vi "Calcudavidflores.vi"() -> ()   [LabVIEW 2018]
uses:
  <vilib>/gmath/NI_Gmath.lvlib
panel:
  out "Ope 3":string
  in  "Numeric":u8
  out "Ope":string
  out "Display 2":string
  out "Ope 2":string
  out "Display":string
  in  "Cluster":T1={"Btn x^2"=FALSE, "Btn Tan -1 3"=FALSE, "Btn Tan -1 2"=FALSE, "Btn ."=FALSE, "Btn 8"=FALSE, "Btn 9"=FALSE, "Btn 7"=FALSE, "Btn 6"=FALSE, "Btn 5"=FALSE, "Btn 4"=FALSE, "Btn 3"=FALSE, "Btn 2"=FALSE, "Btn 1"=FALSE, "Btn 0"=FALSE, "Btn /"=FALSE, "Btn *"=FALSE, "Btn -"=FALSE, "Btn +"=FALSE, "Btn Tan -1"=FALSE, "Btn Cos-1"=FALSE, "Btn Sen -1"=FALSE, "Btn Sqrt"=FALSE, "Btn log"=FALSE, "Btn Tan"=FALSE, "Btn Cos"=FALSE, "Btn Sen"=FALSE, "Btn ="=FALSE, "Btn AC"=FALSE, "Btn Graf"=FALSE, "Btn e^x"=FALSE, "Btn X"=FALSE, "Bot Graficar"=TRUE, "btn grados"=FALSE, "btn radianes"=FALSE}
  out "Display_Calculadora":string
  in  "Display_Graf":string
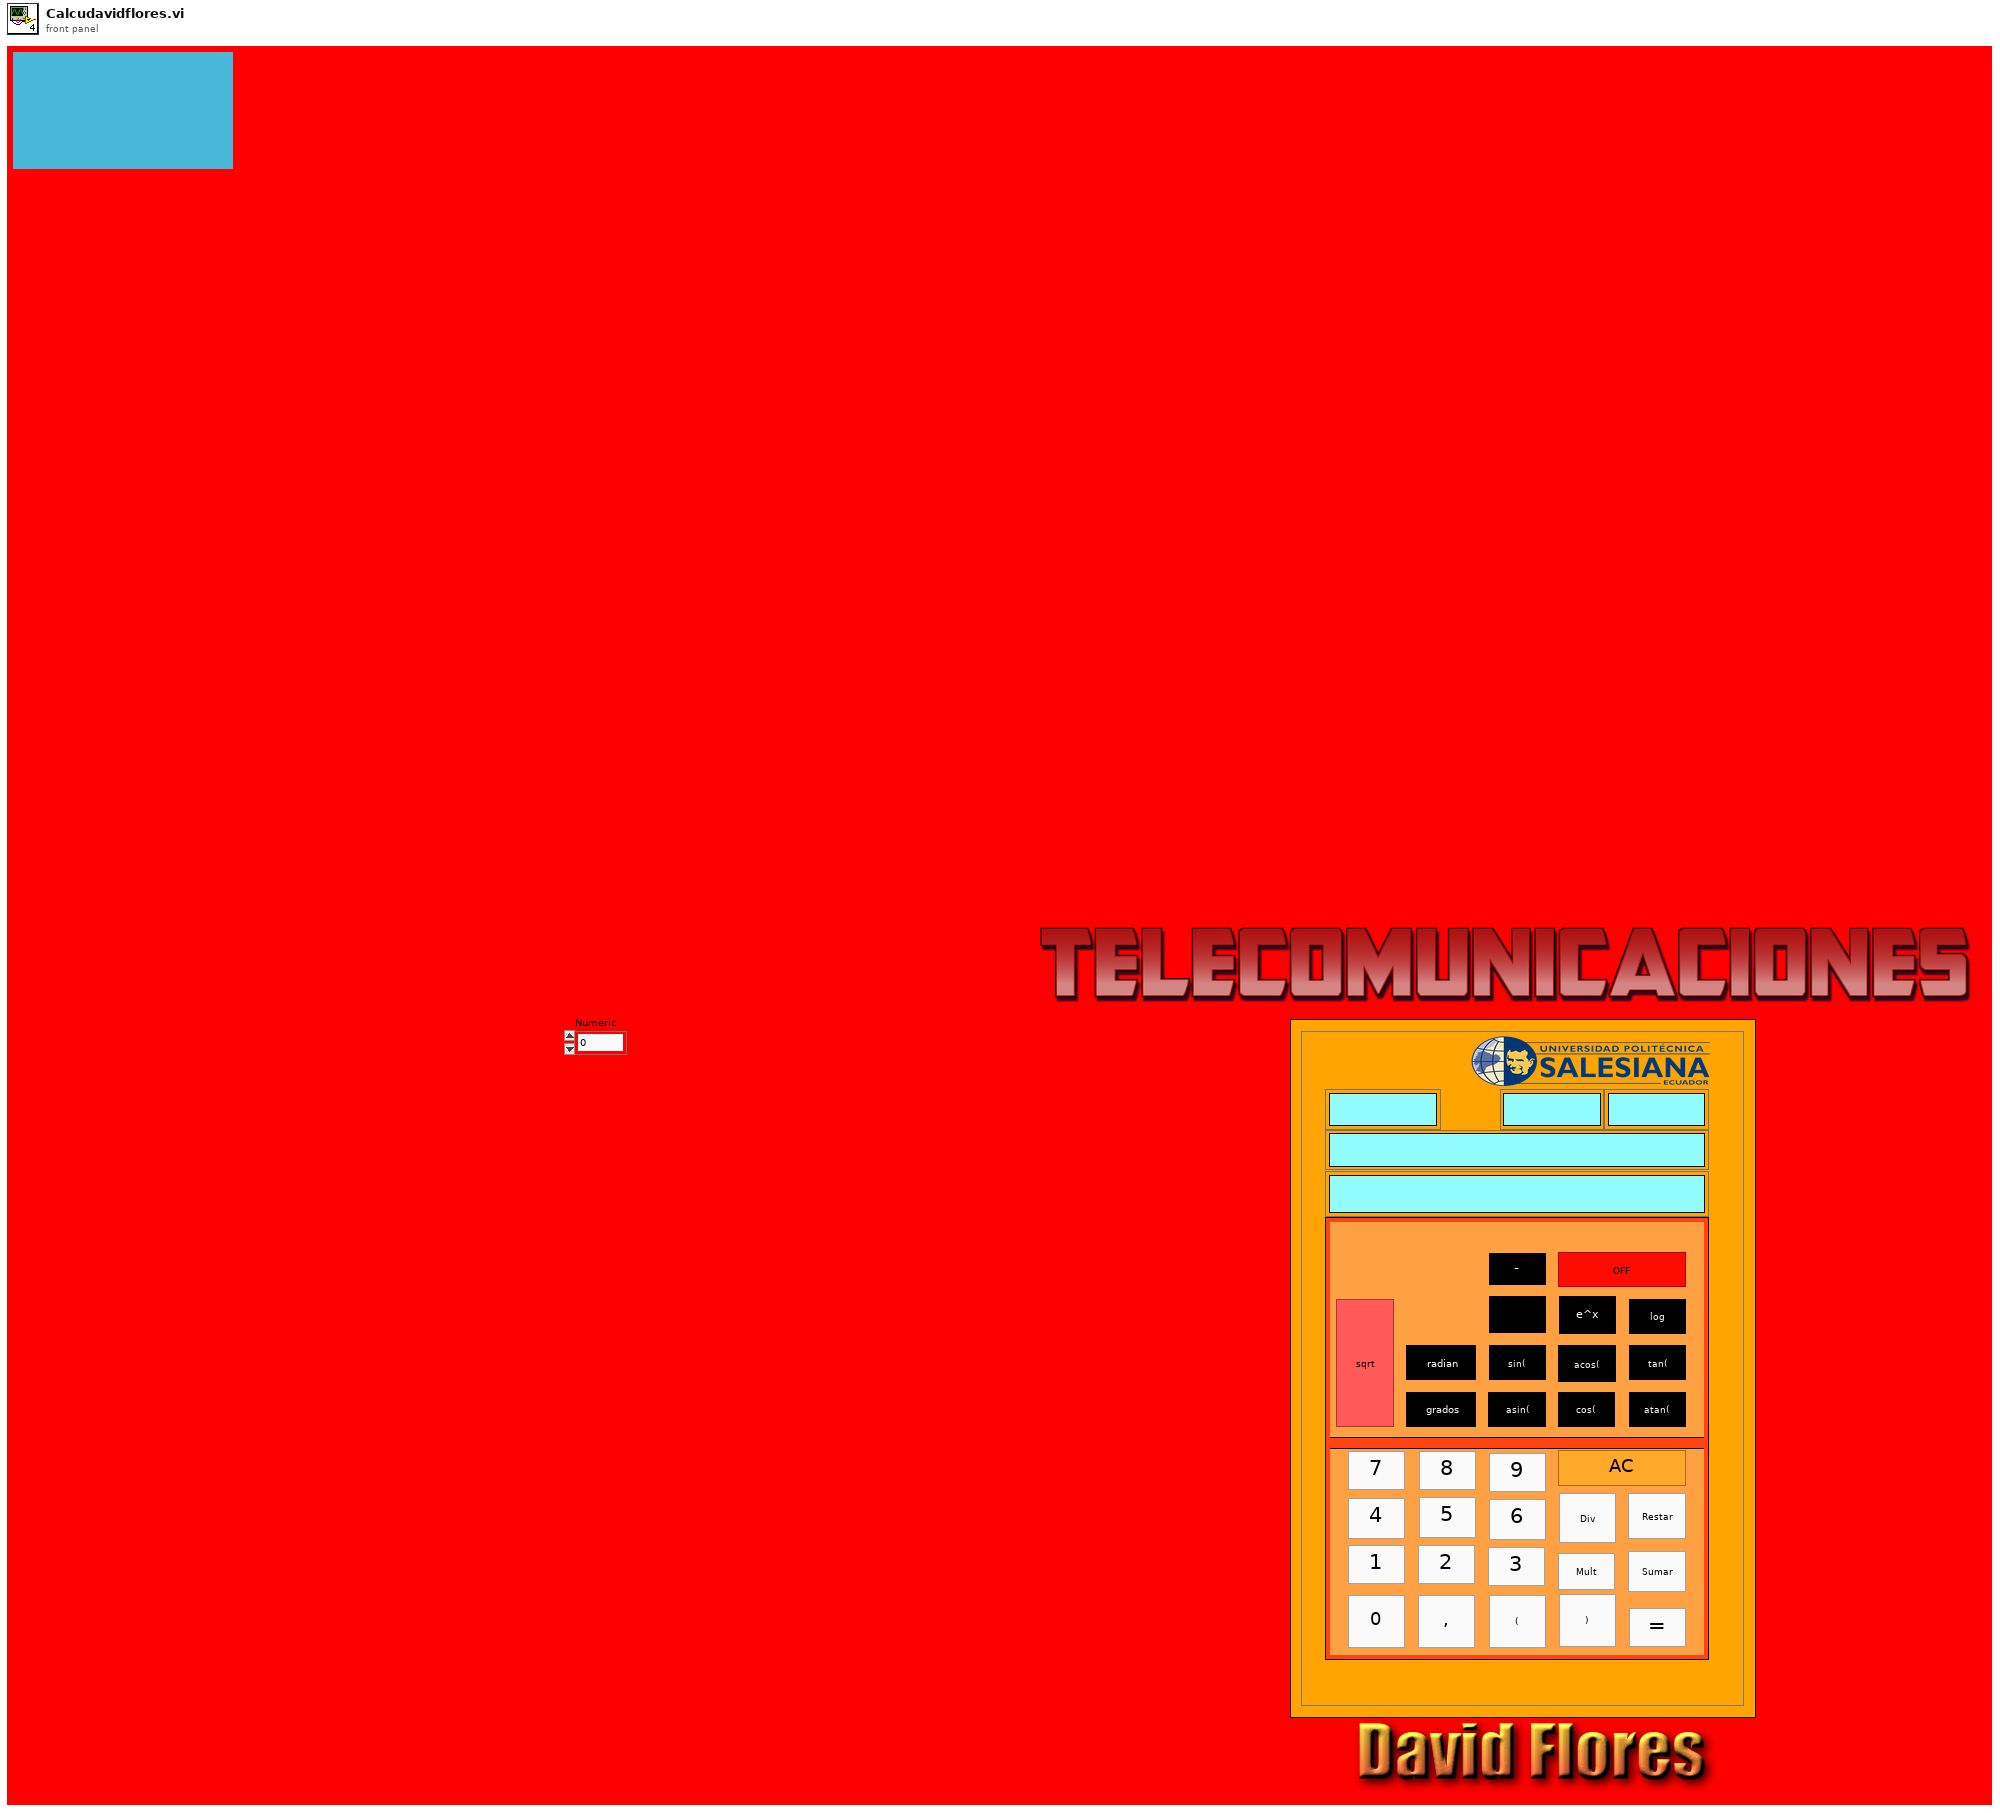
[diagram p1: front panel]
types:
  T1 = cluster{"Btn x^2":bool, "Btn Tan -1 3":bool, "Btn Tan -1 2":bool, "Btn .":bool, "Btn 8":bool, "Btn 9":bool, "Btn 7":bool, "Btn 6":bool, "Btn 5":bool, "Btn 4":bool, "Btn 3":bool, "Btn 2":bool, "Btn 1":bool, "Btn 0":bool, "Btn /":bool, "Btn *":bool, "Btn -":bool, "Btn +":bool, "Btn Tan -1":bool, "Btn Cos-1":bool, "Btn Sen -1":bool, "Btn Sqrt":bool, "Btn log":bool, "Btn Tan":bool, "Btn Cos":bool, "Btn Sen":bool, "Btn =":bool, "Btn AC":bool, "Btn Graf":bool, "Btn e^x":bool, "Btn X":bool, "Bot Graficar":bool, "btn grados":bool, "btn radianes":bool}
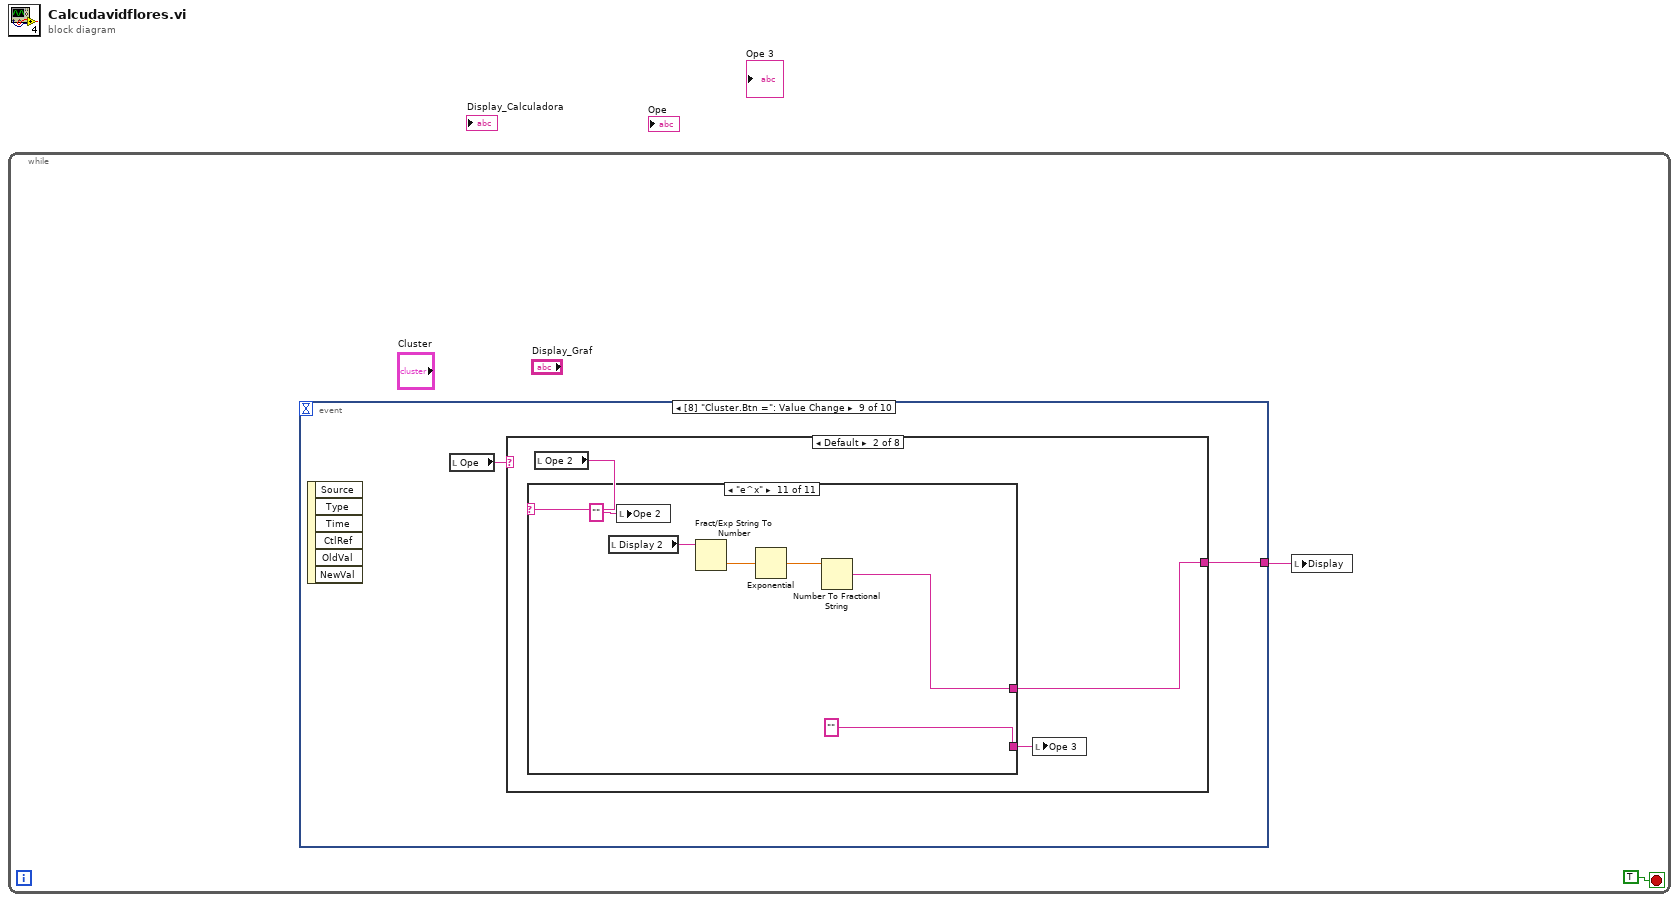
[diagram p0: block diagram]
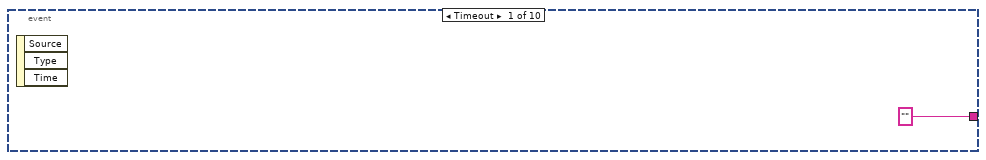
[diagram p2: hidden frame]
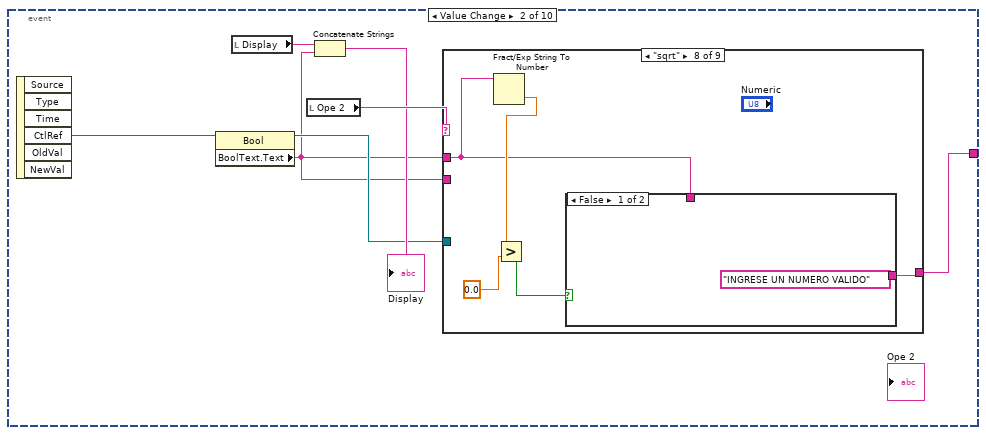
[diagram p3: hidden frame]
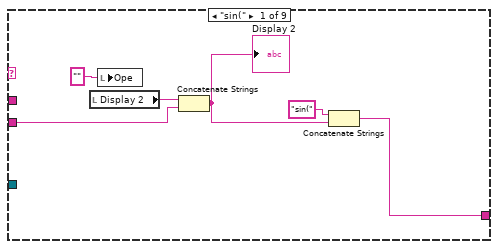
[diagram p4: hidden frame]
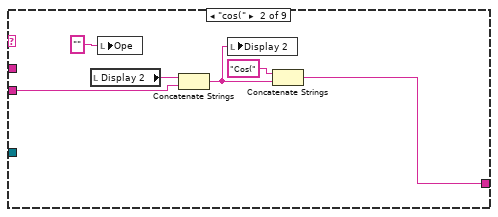
[diagram p5: hidden frame]
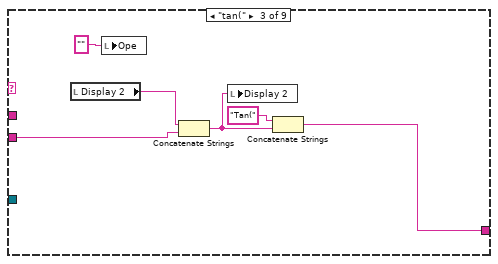
[diagram p6: hidden frame]
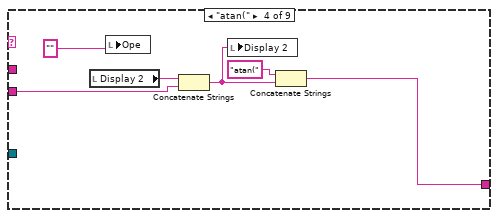
[diagram p7: hidden frame]
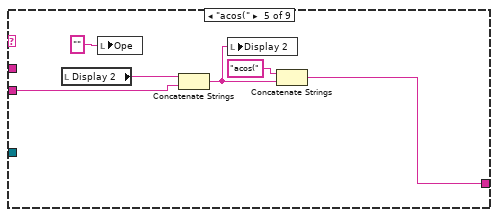
[diagram p8: hidden frame]
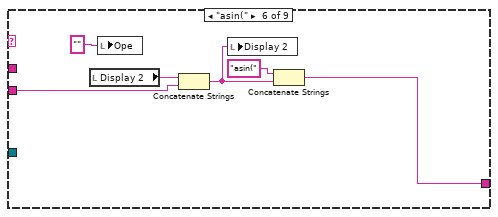
[diagram p9: hidden frame]
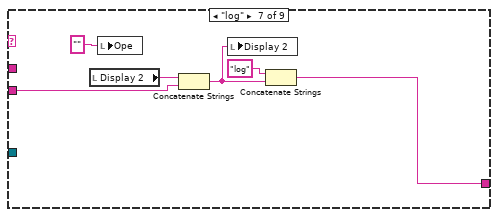
[diagram p10: hidden frame]
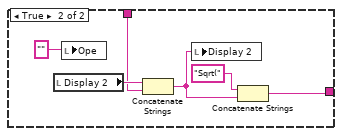
[diagram p11: hidden frame]
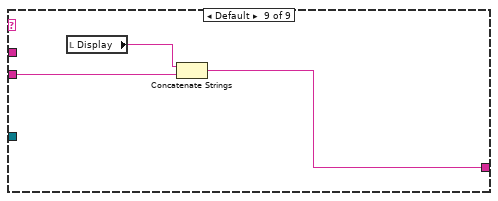
[diagram p12: hidden frame]
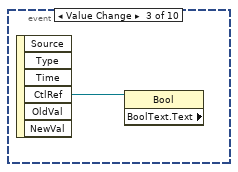
[diagram p13: hidden frame]
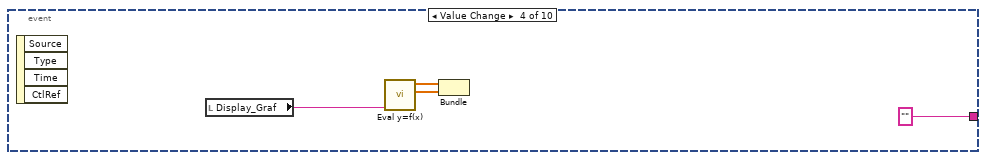
[diagram p14: hidden frame]
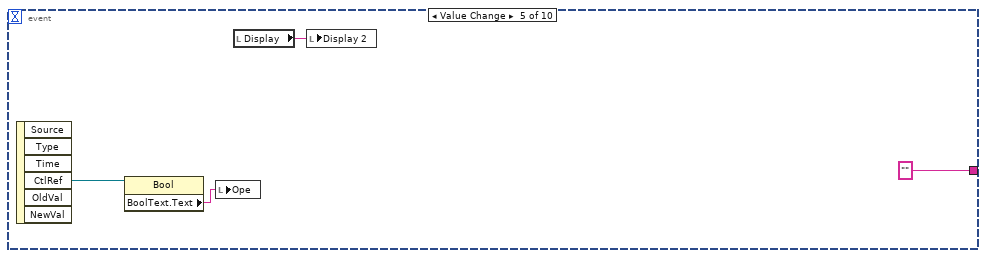
[diagram p15: hidden frame]
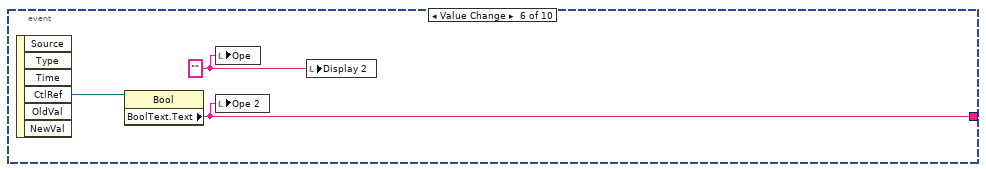
[diagram p16: hidden frame]
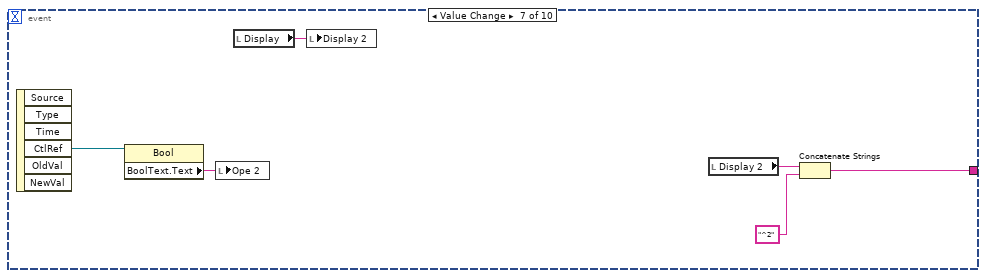
[diagram p17: hidden frame]
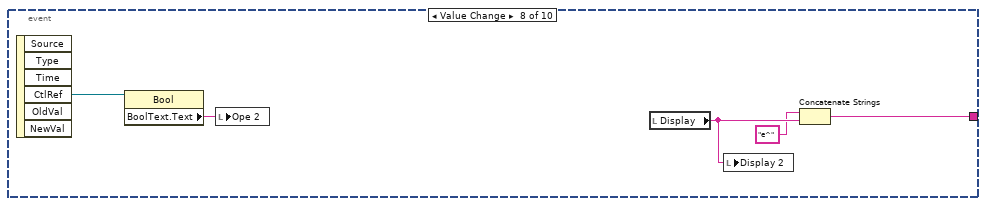
[diagram p18: hidden frame]
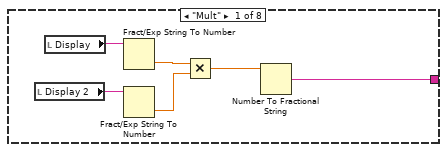
[diagram p19: hidden frame]
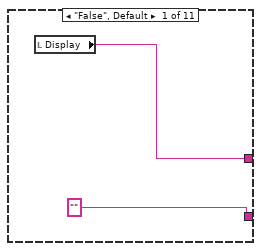
[diagram p20: hidden frame]
diagram:
  n1 = while {
    stop <- TRUE stop-if-true
    n2 = event shown="[8] \"Cluster.Btn =\": Value Change" {
      selector: _ -> [_ _ _ _ _ _ _ _ _ _]
      dyn-events: _ -> [_ _ _ _ _ _ _ _ _ _]
      timeout: _ -> [_ _ _ _ _ _ _ _ _ _]
      tunnel: ["" w8 _ "" "" w77 w82 w87 w91 w212] -> w1
      event Timeout {
        n3 = event-data() -> ()  [unwired: 1 in, 3 out]
      }
      event "Cluster.Btn 0", "Cluster.Btn 1", "Cluster.Btn 2", "Cluster.Btn 3", "Cluster.Btn 4", "Cluster.Btn 5", "Cluster.Btn 6", "Cluster.Btn 7", "Cluster.Btn 8", "Cluster.Btn 9", "Cluster.Btn .", "Cluster.Btn X": Value Change {
        n4 = event-data() -> ("CtlRef"=w10:refnum<vi>)  [unwired: 1 in, 5 out]
        n5 = property class="Bool"(reference=w10) -> (reference out=w5:refnum<vi>, "BoolText.Text"=w4:string)  [unwired: 1 in, 1 out]
        n6 = local read "Display"() -> (w9:string)
        n7 = local read "Ope 2"() -> (w7:string)
        n8 = Concatenate Strings(w9, w4) -> (→"Display":string)
        n9 = case shown="\"sqrt\"" w7 {
          tunnel: w4 -> [w12 w22 w28 w34 w40 w45 w51 _ w67]
          tunnel: [w14 w20 w26 w33 w38 w43 w49 w57 w66] -> w8
          tunnel: w5 -> [_ _ _ _ _ _ _ _ _]
          tunnel: w4 -> [_ _ _ _ _ _ _ w54 _]
          frame "sin(" {
            n10 = local read "Display 2"() -> (w16:string)
            n11 = local write "Ope"("") -> ()
            n12 = Concatenate Strings(w16, w12) -> (w11:string)
            "Display 2" <- w11
            n13 = Concatenate Strings("sin(", w11) -> (w14:string)
          }
          frame "cos(" {
            n14 = local read "Display 2"() -> (w17:string)
            n15 = local write "Ope"("") -> ()
            n16 = Concatenate Strings(w17, w22) -> (w18:string)
            n17 = local write "Display 2"(w18) -> ()
            n18 = Concatenate Strings("Cos(", w18) -> (w20:string)
          }
          frame "tan(" {
            n19 = local read "Display 2"() -> (w23:string)
            n20 = local write "Ope"("") -> ()
            n21 = Concatenate Strings(w23, w28) -> (w24:string)
            n22 = local write "Display 2"(w24) -> ()
            n23 = Concatenate Strings("Tan(", w24) -> (w26:string)
          }
          frame "atan(" {
            n24 = local read "Display 2"() -> (w29:string)
            n25 = local write "Ope"("") -> ()
            n26 = Concatenate Strings(w29, w34) -> (w31:string)
            n27 = local write "Display 2"(w31) -> ()
            n28 = Concatenate Strings("atan(", w31) -> (w33:string)
          }
          frame "acos(" {
            n29 = local read "Display 2"() -> (w35:string)
            n30 = local write "Ope"("") -> ()
            n31 = Concatenate Strings(w35, w40) -> (w36:string)
            n32 = local write "Display 2"(w36) -> ()
            n33 = Concatenate Strings("acos(", w36) -> (w38:string)
          }
          frame "asin(" {
            n34 = local read "Display 2"() -> (w46:string)
            n35 = local write "Ope"("") -> ()
            n36 = Concatenate Strings(w46, w45) -> (w41:string)
            n37 = local write "Display 2"(w41) -> ()
            n38 = Concatenate Strings("asin(", w41) -> (w43:string)
          }
          frame "log" {
            n39 = local read "Display 2"() -> (w52:string)
            n40 = local write "Ope"("") -> ()
            n41 = Concatenate Strings(w52, w51) -> (w47:string)
            n42 = local write "Display 2"(w47) -> ()
            n43 = Concatenate Strings("log", w47) -> (w49:string)
          }
          frame "sqrt" {
            n44 = Fract/Exp String To Number(string=w54) -> (number=w55:dbl)  [unwired: 3 in, 1 out]
            n45 = Greater?(x=w55, y=0.0) -> (0:w56:bool)
            n46 = case shown="False" w56 {
              tunnel: ["INGRESE UN NUMERO VALIDO" w59] -> w57
              tunnel: w54 -> [_ w60]
              frame False {
              }
              frame True {
                n47 = local read "Display 2"() -> (w64:string)
                n48 = local write "Ope"("") -> ()
                n49 = Concatenate Strings(w64, w60) -> (w63:string)
                n50 = local write "Display 2"(w63) -> ()
                n51 = Concatenate Strings("Sqrt(", w63) -> (w59:string)
              }
            }
          }
          frame Default {
            n52 = local read "Display"() -> (w65:string)
            n53 = Concatenate Strings(w65, w67) -> (w66:string)
          }
        }
      }
      event "Cluster.Btn Tan -1 2", "Cluster.Btn Tan -1 3": Value Change {
        n54 = event-data() -> ("CtlRef"=w68:refnum<vi>)  [unwired: 1 in, 5 out]
        n55 = property class="Bool" props=["BoolText", "Text"](reference=w68) -> ()  [unwired: 1 in, 3 out]
      }
      event "Cluster.Bot Graficar": Value Change {
        n56 = event-data() -> ()  [unwired: 1 in, 4 out]
        n57 = local read "Display_Graf"() -> (w69:string)
        n58 = call <vilib>:"Eval y=f(x).vi"("formula"=w69) -> ("Y Values"=w71:dbl[], "X Values"=w72:dbl[])  [unwired: 3 in, 2 out]
        n59 = Bundle("X Values"=w72, "Y Values"=w71) -> ()  [unwired: 1 in, 1 out]
      }
      event "Cluster.Btn *", "Cluster.Btn +", "Cluster.Btn -", "Cluster.Btn /", "Cluster.btn grados", "Cluster.btn radianes": Value Change {
        n60 = event-data() -> ("CtlRef"=w76:refnum<vi>)  [unwired: 1 in, 5 out]
        n61 = property class="Bool"(reference=w76) -> ("BoolText.Text"=w73:string)  [unwired: 1 in, 2 out]
        n62 = local write "Ope"(w73) -> ()
        n63 = local read "Display"() -> (w75:string)
        n64 = local write "Display 2"(w75) -> ()
      }
      event "Cluster.Btn Sen", "Cluster.Btn Cos", "Cluster.Btn Tan", "Cluster.Btn log", "Cluster.Btn Sen -1", "Cluster.Btn Cos-1", "Cluster.Btn Tan -1", "Cluster.Btn Sqrt": Value Change {
        w78 = ""
        n65 = event-data() -> ("CtlRef"=w79:refnum<vi>)  [unwired: 1 in, 5 out]
        n66 = property class="Bool"(reference=w79) -> ("BoolText.Text"=w77:string)  [unwired: 1 in, 2 out]
        n67 = local write "Ope"(w78) -> ()
        n68 = local write "Ope 2"(w77) -> ()
        n69 = local write "Display 2"(w78) -> ()
      }
      event "Cluster.Btn x^2": Value Change {
        n70 = event-data() -> ("CtlRef"=w85:refnum<vi>)  [unwired: 1 in, 5 out]
        n71 = property class="Bool"(reference=w85) -> ("BoolText.Text"=w84:string)  [unwired: 1 in, 2 out]
        n72 = local write "Ope 2"(w84) -> ()
        n73 = local read "Display"() -> (w83:string)
        n74 = local write "Display 2"(w83) -> ()
        n75 = local read "Display 2"() -> (w80:string)
        n76 = Concatenate Strings(w80, "^2") -> (w82:string)
      }
      event "Cluster.Btn e^x": Value Change {
        n77 = event-data() -> ("CtlRef"=w90:refnum<vi>)  [unwired: 1 in, 5 out]
        n78 = property class="Bool"(reference=w90) -> ("BoolText.Text"=w89:string)  [unwired: 1 in, 2 out]
        n79 = local write "Ope 2"(w89) -> ()
        n80 = local read "Display"() -> (w88:string)
        n81 = local write "Display 2"(w88) -> ()
        n82 = Concatenate Strings("e^", w88) -> (w87:string)
      }
      event "Cluster.Btn =": Value Change {
        n83 = event-data() -> ()  [unwired: 1 in, 6 out]
        n84 = local read "Ope"() -> (w92:string)
        n85 = case shown="Default" w92 {
          tunnel: [w95 w100 w170 w177 w182 w189 w197 w205] -> w91
          frame "Mult" {
            n86 = local read "Display 2"() -> (w94:string)
            n87 = local read "Display"() -> (w93:string)
            n88 = Fract/Exp String To Number(string=w93) -> (number=w98:dbl)  [unwired: 3 in, 1 out]
            n89 = Fract/Exp String To Number(string=w94) -> (number=w97:dbl)  [unwired: 3 in, 1 out]
            n90 = Multiply(x=w98, y=w97) -> (x*y=w96:dbl)
            n91 = Number To Fractional String(number=w96) -> (F-format string=w95:string)  [unwired: 3 in]
          }
          frame Default {
            n92 = local read "Ope 2"() -> (w101:string)
            n93 = case shown="\"e^x\"" w101 {
              tunnel: [w103 w107 w112 w118 w124 w130 w136 w142 w149 w163 w168] -> w100
              tunnel: ["" "Radian" "Radian" "Radian" "" "Radian" "Radian" "Radian" "" "" ""] -> w99
              frame "False", Default {
                n94 = local read "Display"() -> (w103:string)
              }
              frame "sin(" {
                n95 = local read "Display 2"() -> (w105:string)
                n96 = local write "Ope 2"("") -> ()
                n97 = Fract/Exp String To Number(string=w105) -> (number=w109:dbl)  [unwired: 3 in, 1 out]
                n98 = Sine(x=w109) -> (sin(x)=w108:dbl)
                n99 = Number To Fractional String(number=w108) -> (F-format string=w107:string)  [unwired: 3 in]
              }
              frame "cos(" {
                n100 = local read "Display 2"() -> (w115:string)
                n101 = local write "Ope 2"("") -> ()
                n102 = Fract/Exp String To Number(string=w115) -> (number=w114:dbl)  [unwired: 3 in, 1 out]
                n103 = Cosine(x=w114) -> (cos(x)=w113:dbl)
                n104 = Number To Fractional String(number=w113) -> (F-format string=w112:string)  [unwired: 3 in]
              }
              frame "tan(" {
                n105 = local read "Display 2"() -> (w121:string)
                n106 = local write "Ope 2"("") -> ()
                n107 = Fract/Exp String To Number(string=w121) -> (number=w120:dbl)  [unwired: 3 in, 1 out]
                n108 = Tangent(1:w120) -> (0:w119:dbl)
                n109 = Number To Fractional String(number=w119) -> (F-format string=w118:string)  [unwired: 3 in]
              }
              frame "log" {
                n110 = local read "Display 2"() -> (w127:string)
                n111 = local write "Ope 2"("") -> ()
                n112 = Fract/Exp String To Number(string=w127) -> (number=w126:dbl)  [unwired: 3 in, 1 out]
                n113 = Logarithm Base 10(1:w126) -> (0:w125:dbl)
                n114 = Number To Fractional String(number=w125) -> (F-format string=w124:string)  [unwired: 3 in]
              }
              frame "asin(" {
                n115 = local read "Display 2"() -> (w133:string)
                n116 = local write "Ope 2"("") -> ()
                n117 = Fract/Exp String To Number(string=w133) -> (number=w132:dbl)  [unwired: 3 in, 1 out]
                n118 = Inverse Sine(1:w132) -> (0:w131:dbl)
                n119 = Number To Fractional String(number=w131) -> (F-format string=w130:string)  [unwired: 3 in]
              }
              frame "acos(" {
                n120 = local read "Display 2"() -> (w139:string)
                n121 = local write "Ope 2"("") -> ()
                n122 = Fract/Exp String To Number(string=w139) -> (number=w138:dbl)  [unwired: 3 in, 1 out]
                n123 = Inverse Cosine(1:w138) -> (0:w137:dbl)
                n124 = Number To Fractional String(number=w137) -> (F-format string=w136:string)  [unwired: 3 in]
              }
              frame "atan(" {
                n125 = local read "Display 2"() -> (w145:string)
                n126 = local write "Ope 2"("") -> ()
                n127 = Fract/Exp String To Number(string=w145) -> (number=w144:dbl)  [unwired: 3 in, 1 out]
                n128 = Inverse Tangent(1:w144) -> (0:w143:dbl)
                n129 = Number To Fractional String(number=w143) -> (F-format string=w142:string)  [unwired: 3 in]
              }
              frame "sqrt" {
                n130 = local read "Display 2"() -> (w151:string)
                n131 = local write "Ope 2"("") -> ()
                n132 = Fract/Exp String To Number(string=w151) -> (number=w148:dbl)  [unwired: 3 in, 1 out]
                n133 = Less?(x=w148, y=0.0) -> (x < y?=w150:bool)
                n134 = case shown="True" w150 {
                  tunnel: [w155 "ERROR"] -> w149
                  frame False {
                    n135 = local read "Display 2"() -> (w153:string)
                    n136 = Fract/Exp String To Number(string=w153) -> (number=w154:dbl)  [unwired: 3 in, 1 out]
                    n137 = Square Root(x=w154) -> (sqrt(x)=w156:dbl)
                    n138 = Number To Fractional String(number=w156) -> (F-format string=w155:string)  [unwired: 3 in]
                  }
                  frame True {
                  }
                }
              }
              frame "X^2" {
                n139 = local read "Display 2"() -> (w159:string)
                n140 = local write "Ope 2"("") -> ()
                n141 = Fract/Exp String To Number(string=w159) -> (number=w161:dbl)  [unwired: 3 in, 1 out]
                n142 = Square(x=w161) -> (x^2=w160:dbl)
                n143 = Number To Fractional String(number=w160) -> (F-format string=w163:string)  [unwired: 3 in]
              }
              frame "e^x" {
                n144 = local read "Display 2"() -> (w169:string)
                n145 = local write "Ope 2"("") -> ()
                n146 = Fract/Exp String To Number(string=w169) -> (number=w166:dbl)  [unwired: 3 in, 1 out]
                n147 = Exponential(1:w166) -> (0:w165:dbl)
                n148 = Number To Fractional String(number=w165) -> (F-format string=w168:string)  [unwired: 3 in]
              }
            }
            n149 = local write "Ope 3"(w99) -> ()
          }
          frame "Sumar" {
            n150 = local read "Display 2"() -> (w173:string)
            n151 = local read "Display"() -> (w175:string)
            n152 = Fract/Exp String To Number(string=w175) -> (number=w174:dbl)  [unwired: 3 in, 1 out]
            n153 = Fract/Exp String To Number(string=w173) -> (number=w172:dbl)  [unwired: 3 in, 1 out]
            n154 = Add(x=w174, y=w172) -> (x+y=w171:dbl)
            n155 = Number To Fractional String(number=w171) -> (F-format string=w170:string)  [unwired: 3 in]
          }
          frame "Div" {
            n156 = local read "Display"() -> (w176:string)
            n157 = local read "Display 2"() -> (w181:string)
            n158 = Fract/Exp String To Number(string=w181) -> (number=w180:dbl)  [unwired: 3 in, 1 out]
            n159 = Fract/Exp String To Number(string=w176) -> (number=w179:dbl)  [unwired: 3 in, 1 out]
            n160 = Divide(x=w180, y=w179) -> (x/y=w178:dbl)
            n161 = Number To Fractional String(number=w178) -> (F-format string=w177:string)  [unwired: 3 in]
          }
          frame "Restar" {
            n162 = local read "Display 2"() -> (w187:string)
            n163 = local read "Display"() -> (w185:string)
            n164 = Fract/Exp String To Number(string=w187) -> (number=w186:dbl)  [unwired: 3 in, 1 out]
            n165 = Fract/Exp String To Number(string=w185) -> (number=w184:dbl)  [unwired: 3 in, 1 out]
            n166 = Subtract(x=w186, y=w184) -> (x-y=w183:dbl)
            n167 = Number To Fractional String(number=w183) -> (F-format string=w182:string)  [unwired: 3 in]
          }
          frame "grados" {
            n168 = local read "Display 2"() -> (w195:string)
            n169 = Fract/Exp String To Number(string=w195) -> (number=w193:dbl)  [unwired: 3 in, 1 out]
            n170 = Multiply(x=w193, y=180) -> (x*y=w192:dbl)
            n171 = Divide(x=w192, y=3.1416) -> (x/y=w190:dbl)
            n172 = Number To Fractional String(number=w190) -> (F-format string=w189:string)  [unwired: 3 in]
            n173 = local write "Ope 3"("") -> ()
          }
          frame "radian" {
            n174 = local read "Display 2"() -> (w203:string)
            n175 = Fract/Exp String To Number(string=w203) -> (number=w201:dbl)  [unwired: 3 in, 1 out]
            n176 = Multiply(x=w201, y=3.1596) -> (x*y=w199:dbl)
            n177 = Divide(x=w199, y=180) -> (x/y=w198:dbl)
            n178 = Number To Fractional String(number=w198) -> (F-format string=w197:string)  [unwired: 3 in]
            n179 = local write "Ope 3"("") -> ()
          }
          frame "degr" {
            n180 = local read "Display 2"() -> (w211:string)
            n181 = Fract/Exp String To Number(string=w211) -> (number=w209:dbl)  [unwired: 3 in, 1 out]
            n182 = Multiply(x=w209, y=200) -> (x*y=w207:dbl)
            n183 = Divide(x=w207, y=180) -> (x/y=w206:dbl)
            n184 = Number To Fractional String(number=w206) -> (F-format string=w205:string)  [unwired: 3 in]
            n185 = local write "Ope 3"("") -> ()
          }
        }
      }
      event "Cluster.Btn AC": Value Change {
        w212 = ""
        n186 = event-data() -> ()  [unwired: 1 in, 6 out]
        n187 = local write "Ope 2"(w212) -> ()
        n188 = local write "Ope"(w212) -> ()
        n189 = local write "Display_Graf"(w212) -> ()
        n190 = local write "Display 2"(w212) -> ()
        n191 = local write "Ope 3"(w212) -> ()
      }
    }
    n192 = local write "Display"(w1) -> ()
  }
